vi "Apply.vi"(8 "error in (no error)":errorcluster, 11 "DIO DAQmx PWM CFG in":refnum<class "DIO DAQmx PWM CFG.lvclass">) -> (0 "error out":errorcluster, 3 "DIO DAQmx PWM CFG out":refnum<class "DIO DAQmx PWM CFG.lvclass">)   [LabVIEW 2023, in "DIO DAQmx PWM CFG.lvclass"]
uses:
  DIO DAQmx PWM CFG.lvclass
  DIO DAQmx PWM CFG.lvclass/DIO DAQmx PWM CFG.ctl
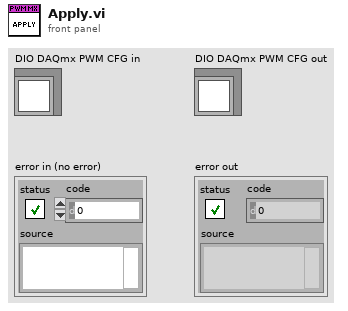
[diagram p1: front panel]
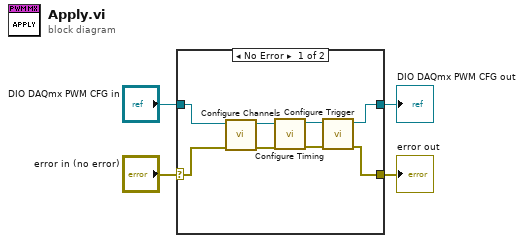
[diagram p0: block diagram]
diagram:
  n1 = case shown="No Error" "error in (no error)" {
    selector: "error in (no error)" -> [w7 w13]
    tunnel: "DIO DAQmx PWM CFG in" -> [w8 w14]
    tunnel: [w6 w13] -> w2
    tunnel: [w5 w14] -> w1
    frame No Error {
      n2 = call-dynamic "Configure Channels.vi"("error in (no error)"=w7, "DIO DAQmx PWM CFG in"=w8) -> ("error out"=w11:errorcluster, "DIO DAQmx PWM CFG out"=w12:refnum<class "DIO DAQmx PWM CFG.lvclass">)  [unwired: 8 in]
      n3 = call-dynamic "Configure Timing.vi"("error in (no error)"=w11, "DAQmx Base CFG in"=w12) -> ("error out"=w9:errorcluster, "DAQmx Base CFG out"=w10:refnum<class "DIO DAQmx PWM CFG.lvclass">)  [unwired: 8 in]
      n4 = call-dynamic "Configure Trigger.vi"("error in (no error)"=w9, "DAQmx Base CFG in"=w10) -> ("error out"=w6:errorcluster, "DAQmx Base CFG out"=w5:refnum<class "DIO DAQmx PWM CFG.lvclass">)  [unwired: 8 in]
    }
    frame Error {
    }
  }
  "error out" <- w2
  "DIO DAQmx PWM CFG out" <- w1
